vi "Delete EST Loops.vi"(8 "error in (no error)":errorcluster, 11 "Main Sequence in":refnum<class "Main Sequence.lvclass">) -> (0 "error out":errorcluster, 3 "Main Sequence out":refnum<class "Main Sequence.lvclass">)   [LabVIEW 2025, in "Main Sequence.lvclass"]
doc: "Find the EST pieces that are in the template and need to be removed. Delete."
uses:
  Main Sequence.lvclass
  Structures/Structures.lvclass/Structures.ctl
  Structures/Read Structure.vi
  Main Sequence.lvclass/Main Sequence.ctl
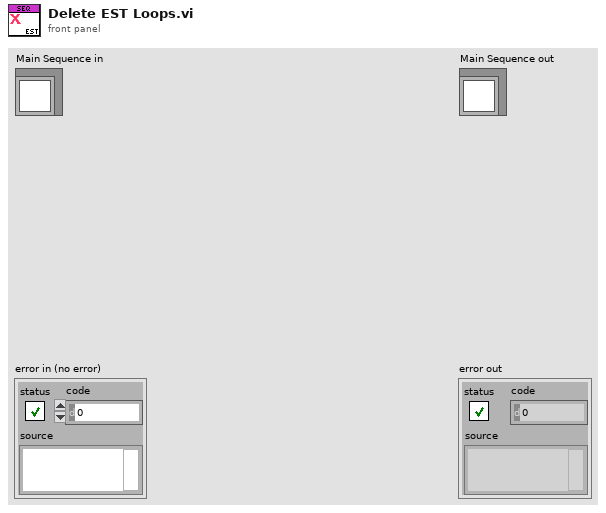
[diagram p1: front panel]
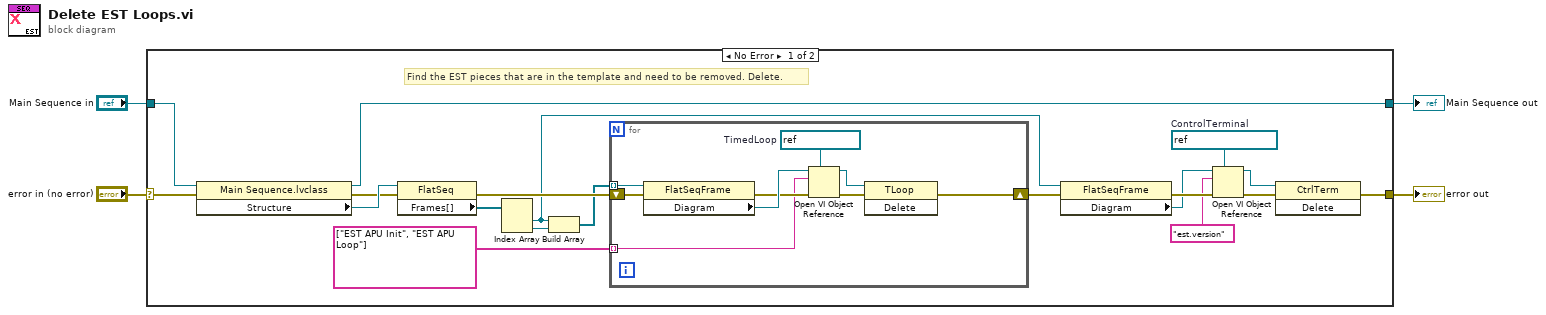
[diagram p0: block diagram]
diagram:
  n1 = case shown="No Error" "error in (no error)" {
    selector: "error in (no error)" -> [w21 w34]
    tunnel: [w6 w34] -> w3
    tunnel: [w22 w33] -> w1
    tunnel: "Main Sequence in" -> [w23 w33]
    frame No Error {
      w9 = refnum<vi> refnum  # ControlTerminal
      # "Find the EST pieces that are in the template and need to be removed. Delete."
      n2 = property class="Main Sequence.lvclass"(reference=w23, error in=w21) -> (reference out=w22:refnum<class "Main Sequence.lvclass">, error out=w19:errorcluster, "Structure"=w20:refnum<vi>)
      n3 = property class="FlatSeq"(reference=w20, error in=w19) -> (error out=w18:errorcluster, "Frames[]"=w16:refnum<vi>[])  [unwired: 1 out]
      n4 = Index Array(array=w16) -> (element #1=w13:refnum<vi>, element #2=w15:refnum<vi>)  [unwired: 2 in]
      n5 = Build Array(w13, w15) -> (w14:refnum<vi>[])
      n6 = for {
        tunnel: w14 -> [w31] mode=indexing
        shift-right: [w24] -> w12
        shift-left: w18 -> [w32]
        tunnel: string[] ["EST APU Init", "EST APU Loop"] -> [w27] mode=indexing
        w29 = refnum<vi> refnum  # TimedLoop
        n7 = property class="FlatSeqFrame"(reference=w31, error in=w32) -> (error out=w28:errorcluster, "Diagram"=w30:refnum<vi>)  [unwired: 1 out]
        n8 = Open VI Object Reference(7:w29, 8:w28, 10:w27, 11:w30) -> (0:w25:errorcluster, 3:w26:refnum<vi>)
        n9 = invoke class="TLoop" method="Delete"(reference=w26, error in=w25) -> (error out=w24:errorcluster)  [unwired: 1 in, 2 out]
      }
      n10 = property class="FlatSeqFrame"(reference=w13, error in=w12) -> (error out=w11:errorcluster, "Diagram"=w10:refnum<vi>)  [unwired: 1 out]
      n11 = Open VI Object Reference(7:w9, 8:w11, 10:"est.version", 11:w10) -> (0:w8:errorcluster, 3:w7:refnum<vi>)
      n12 = invoke class="CtrlTerm" method="Delete"(reference=w7, error in=w8) -> (error out=w6:errorcluster)  [unwired: 1 in, 2 out]
    }
    frame Error {
    }
  }
  "error out" <- w3
  "Main Sequence out" <- w1
